vi "ProcessTTRecTH260T3.vi"(8 "oflcorr_in":u64, 11 "rawbits":u32) -> (0 "markercode":u32, 1 "is_marker":bool, 2 "channel":u32, 3 "dtime":u32, 4 "oflcorr_out":u64, 5 "numsync":u64, 7 "is_photon":bool)   [LabVIEW 2017]
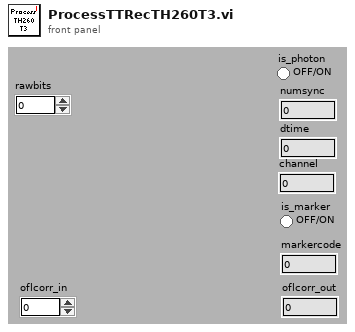
[diagram p1: front panel]
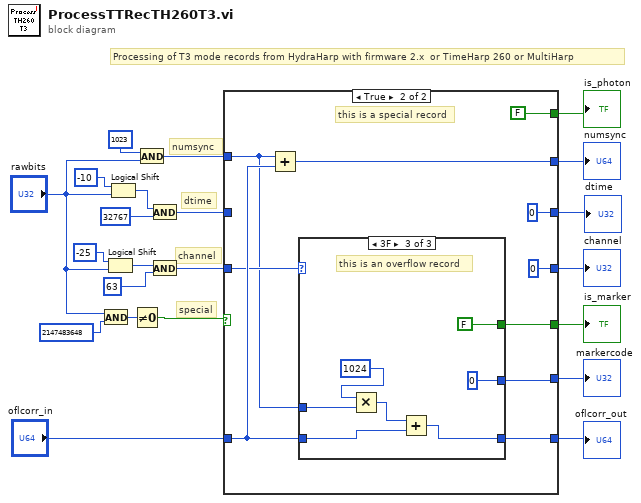
[diagram p0: block diagram]
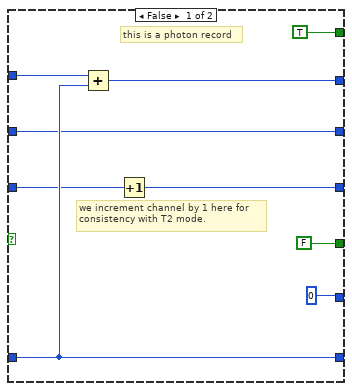
[diagram p2: hidden frame]
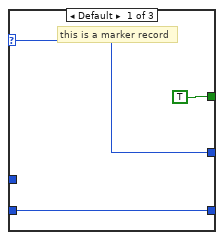
[diagram p3: hidden frame]
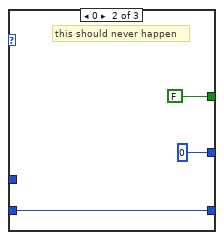
[diagram p4: hidden frame]
diagram:
  # "special"
  # "Processing of T3 mode records from HydraHarp with firmware 2.x  or TimeHarp 260 or MultiHarp"
  # "dtime"
  # "channel"
  # "numsync"
  n1 = And(x="rawbits", y=u32 2147483648 ("x")) -> (x .and. y?=w5:u32)
  n2 = Logical Shift(y=-25, x="rawbits") -> (x << y=w15:u32)
  n3 = Logical Shift(y=-10, x="rawbits") -> (x << y=w18:u32)
  n4 = Not Equal To 0?(x=w5) -> (x != 0?=w2:bool)
  n5 = And(x=u32 1023, y="rawbits") -> (x .and. y?=w20:u32)
  n6 = And(x=w18, y=u32 32767 ("x")) -> (x .and. y?=w16:u32)
  n7 = And(x=w15, y=u32 63 ("x")) -> (x .and. y?=w1:u32)
  n8 = case shown="True" w2 {
    tunnel: w20 -> [w25 w33]
    tunnel: "oflcorr_in" -> [w28 w38]
    tunnel: [w28 w37] -> w12
    tunnel: [FALSE w35] -> w10
    tunnel: [u32 0 w36] -> w11
    tunnel: [TRUE FALSE] -> w8
    tunnel: w16 -> [w26 _]
    tunnel: [w27 w41] -> w7
    tunnel: [w26 u32 0] -> w6
    tunnel: [w23 u32 0] -> w9
    tunnel: w1 -> [w24 w34]
    frame False {
      # "we increment channel by 1 here for\nconsistency with T2 mode."
      # "this is a photon record"
      n9 = Add(x=w25, y=w28) -> (x+y=w27:u64)
      n10 = Increment(x=w24) -> (x+1=w23:u32)
    }
    frame True {
      # "this is a special record"
      n11 = Add(x=w33, y=w38) -> (x+y=w41:u64)
      n12 = case shown="3F" w34 {
        selector: w34 -> [w42 _ _]
        tunnel: w38 -> [w44 w45 w54]
        tunnel: [w44 w45 w53] -> w37
        tunnel: [TRUE FALSE FALSE] -> w35
        tunnel: [w42 u32 0 u32 0] -> w36
        tunnel: w33 -> [_ _ w48]
        frame Default {
          # "this is a marker record"
        }
        frame 0 {
          # "this should never happen"
        }
        frame 63 {
          # "this is an overflow record"
          n13 = Multiply(x=u64 1024, y=w48) -> (x*y=w50:u64)
          n14 = Add(x=w50, y=w54) -> (x+y=w53:u64)
        }
      }
    }
  }
  "channel" <- w9
  "numsync" <- w7
  "is_photon" <- w8
  "markercode" <- w11
  "is_marker" <- w10
  "oflcorr_out" <- w12
  "dtime" <- w6
